vi "Test Thorlabs Module.vi"() -> ()   [LabVIEW 2018]
panel:
  out "#Blines":dbl
  out "Data Out":sgl[][](array[numeric])
  in  "acquire":T1(ring)=enum."Acquire RAW"
  in  "start":T1(ring)=enum."Start Acquire Raw"
  in  "configure":T1(ring)=enum."Configure"
  in  "Objective":u16(ring)=1 items=["5X LKM05", "10X LKM10", "20X LKM20", "10X LSM02"]
  in  "ROI Parameters":T2={"ROI (mm)"={"X (mm)"=1.0, "Y (mm)"=1.0}, "Shift (mm)"={"Xshift (mm)"=0.0, "Yshift (mm)"=0.0}}
  in  "Scan Parameters":T3={"# Scan"={"#Ascan"=400, "#Bscan"=400}, "# Rpt"={"#ARpt"=1, "#BRpt"=1}, "Aline Rate"=2, "# Extra"={"# ARpt_extra"=5, "#Brtn_extra"=60}} {"Aline Rate" items=["76 KHz", "146 KHz", "76 KHz", "28 KHz", "10 KHz"]}
  out "unit error":errorcluster
  out "Raw Data Out":u16[][](array[numeric])
  in  "error constant":errorcluster
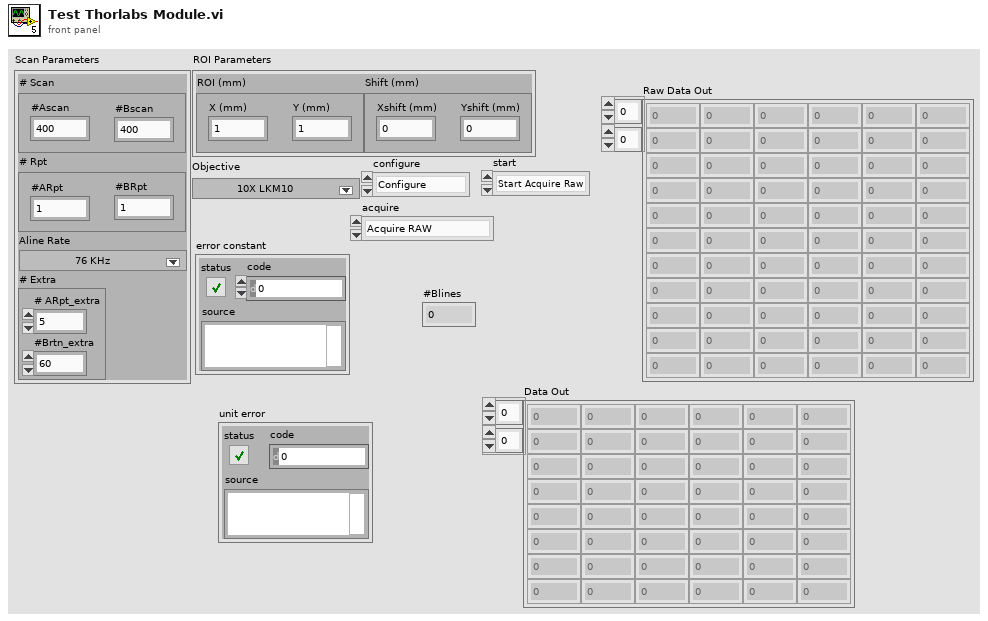
[diagram p1: front panel]
types:
  T1 = enum16{"Init", "Configure", "Configure Data", "Generate Scan Pattern", "Start Acquire Raw", "Start Acquire Data", "Acquire RAW", "Acquire Data", "Stop Acquire", "Uninit"}
  T2 = cluster{"ROI (mm)":cluster{"X (mm)":dbl, "Y (mm)":dbl}, "Shift (mm)":cluster{"Xshift (mm)":sgl, "Yshift (mm)":sgl}}
  T3 = cluster{"# Scan":cluster{"#Ascan":i32, "#Bscan":i32}, "# Rpt":cluster{"#ARpt":i32, "#BRpt":i32}, "Aline Rate":u16, "# Extra":cluster{"# ARpt_extra":i32, "#Brtn_extra":i32}}
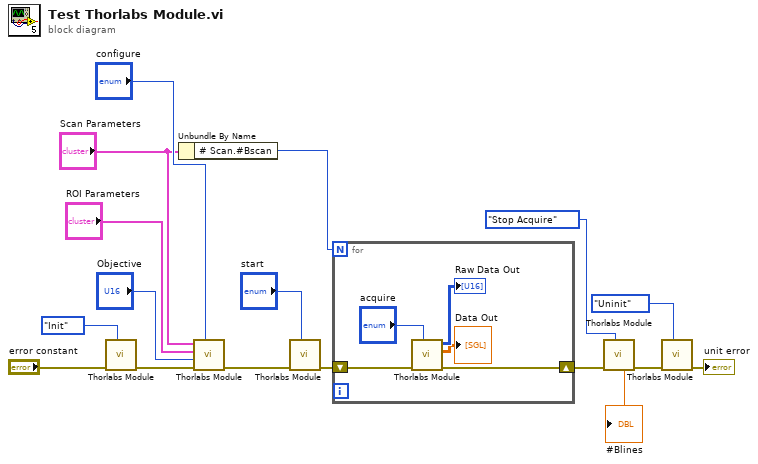
[diagram p0: block diagram]
diagram:
  n1 = call "Thorlabs Module.vi"("Actions"=T1."Init", "error in"="error constant") -> ("error out"=w16:errorcluster)  [unwired: 6 in, 3 out]
  n2 = Unbundle By Name("Scan Parameters") -> ("# Scan.#Bscan"=w2:i32)
  n3 = call "Thorlabs Module.vi"("Actions"="configure", "error in"=w16, "Objective"="Objective", "ROI Parameters"="ROI Parameters", "Scan Parameters"="Scan Parameters") -> ("error out"=w15:errorcluster)  [unwired: 3 in, 3 out]
  n4 = call "Thorlabs Module.vi"("Actions"="start", "error in"=w15) -> ("error out"=w14:errorcluster)  [unwired: 6 in, 3 out]
  n5 = for {
    N: w2 -> [_]
    shift-right: [w21] -> w13
    shift-left: w14 -> [w22]
    n6 = call "Thorlabs Module.vi"("Actions"="acquire", "error in"=w22) -> ("error out"=w21:errorcluster, "Data Out"=→"Data Out":sgl[][], "Raw Data Out"=→"Raw Data Out":u16[][])  [unwired: 6 in, 1 out]
  }
  n7 = call "Thorlabs Module.vi"("Actions"=T1."Stop Acquire", "error in"=w13) -> ("error out"=w12:errorcluster, "#Blines"=→"#Blines":dbl)  [unwired: 6 in, 2 out]
  n8 = call "Thorlabs Module.vi"("Actions"=T1."Uninit", "error in"=w12) -> ("error out"=→"unit error":errorcluster)  [unwired: 6 in, 3 out]
